vi "叶绿素a_获取温度和叶绿素值.vi"(8 "error in (no error)":errorcluster caption="错误输入（无错误）", 11 "MB session in":refnum<class "MB_Master.lvclass">) -> (0 "error out":errorcluster caption="错误输出", 2 "输出值":cluster{"温度测量值":sgl, "叶绿素测量值":sgl, "错误标志":u16} {"错误标志" items=["NO Error"=0, "刷子没到位"=255]}, 3 "MB session out":refnum<class "MB_Master.lvclass">)   [LabVIEW 2016, in "斯坦道多参数.lvlib"]
uses:
  <vilib>/Plasmionique/MB Master/MB_Master/MB_Master.lvclass
  <vilib>/Plasmionique/MB Master/MB Master.lvlib
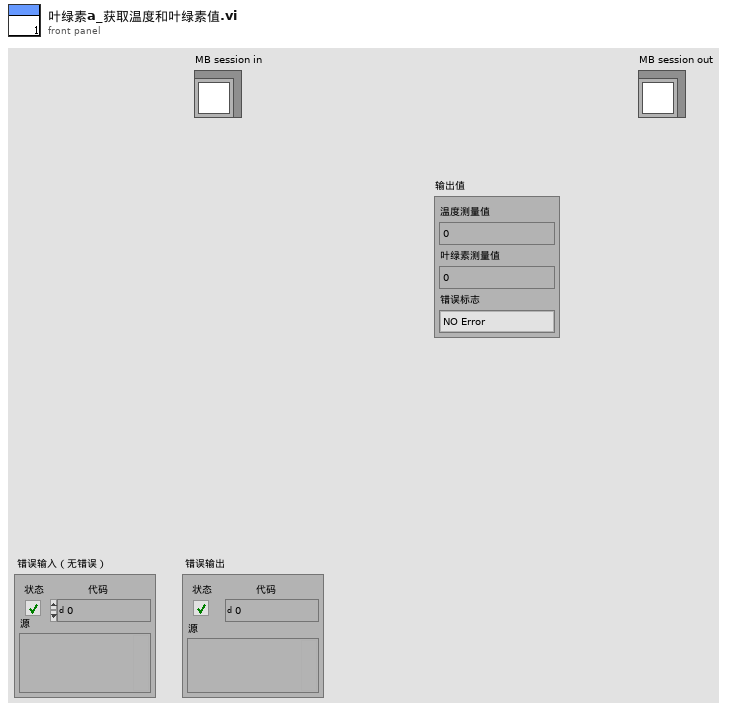
[diagram p1: front panel]
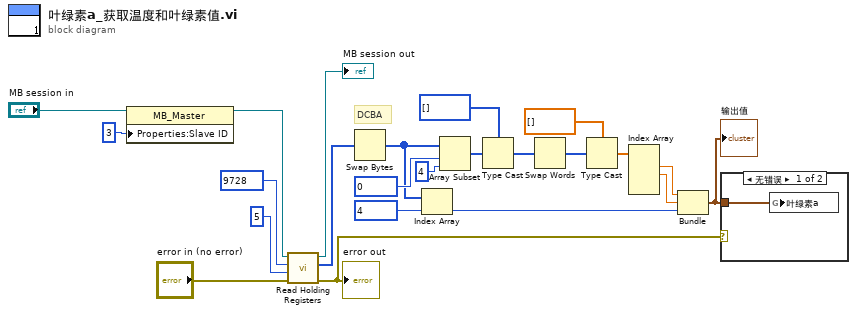
[diagram p0: block diagram]
diagram:
  # "DCBA"
  n1 = property class="MB_Master"(reference="MB session in", "Properties:Slave ID"=u16 3 ("y")) -> (reference out=w11:refnum<class "MB_Master.lvclass">)  [unwired: 1 in, 1 out]
  n2 = call <vilib>:"Read Holding Registers.vi"("error in (no error)"="error in (no error)", "quantity"=u16 5, "starting address"=u16 9728, "MB session in"=w11) -> ("error out"=w4:errorcluster, "Registers"=w7:u16[], "MB session out"=→"MB session out":refnum<class "MB_Master.lvclass">)  [unwired: 5 in]
  "error out" <- w4
  n3 = Swap Bytes(anything=w7) -> (byte swapped=w6:u16[])
  n4 = Index Array(array=w6, index=u16 4 ("starting address")) -> (element=w8:u16)
  n5 = Array Subset(array=w6, index=u16 0 ("starting address"), length=4 ("长度")) -> (w5:u16[])
  n6 = Type Cast(type=u32[] [] ("数组 2"), x=w5) -> (*(type *) &x=w18:u32[])
  n7 = Swap Words(1:w18) -> (0:w20:u32[])
  n8 = Type Cast(type=sgl[] [] ("数组 2"), x=w20) -> (*(type *) &x=w16:sgl[])
  n9 = Index Array(array=w16) -> (element #1=w15:sgl, element #2=w14:sgl)  [unwired: 4 in, 2 out]
  n10 = Bundle("数值"=w15, "数值"=w14, w8) -> (w3:cluster{"数值":sgl, "数值":sgl, u16})  [unwired: 1 in]
  "输出值" <- w3
  n11 = case shown="无错误" w4 {
    tunnel: w3 -> [w24 _]
    frame No Error {
      n12 = global write "禹山过程全局变量.vi" "叶绿素a"(w24) -> ()
    }
    frame Error {
    }
  }
